vi "Get Sample Rate.vi"(8 "error in (no error)":errorcluster, 11 "Impulse Manager in":refnum<class "Impulse Manager.lvclass">) -> (0 "error out":errorcluster, 2 "Sample Rate":i32, 3 "Impulse Manager out":refnum<class "Impulse Manager.lvclass">)   [LabVIEW 2013, in "Impulse Manager.lvclass"]
uses:
  Impulse Manager.lvclass
  Impulse Manager.lvclass/Impulse Manager.ctl
  Impulse Data/Impulse Data.lvclass
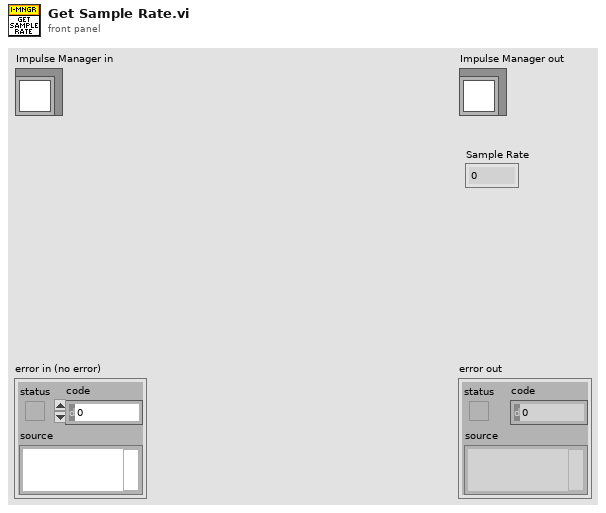
[diagram p1: front panel]
types:
  T1 = typedef "Impulse Data.lvclass/Instance handle.ctl" = refnum<data-value>
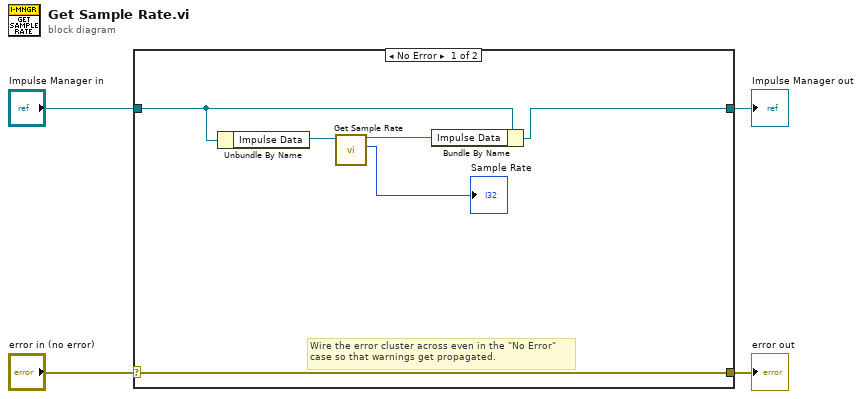
[diagram p0: block diagram]
diagram:
  n1 = case shown="No Error" "error in (no error)" {
    selector: "error in (no error)" -> [w10 w12]
    tunnel: [w10 w12] -> w3
    tunnel: [w7 w11] -> w1
    tunnel: "Impulse Manager in" -> [w8 w11]
    frame No Error {
      # "Wire the error cluster across even in the \"No Error\"\ncase so that warnings get propagated."
      n2 = Unbundle By Name(w8) -> ("Impulse Data"=w9:T1)
      n3 = call "Get Sample Rate.vi"("Reference in"=w9) -> ("Sample Rate"=→"Sample Rate":i32, "Reference out"=w6:T1)  [unwired: 8 in, 1 out]
      n4 = Bundle By Name(cluster=w8, "Impulse Data"=w6) -> (w7:refnum<class "Impulse Manager.lvclass">)
    }
    frame Error {
    }
  }
  "error out" <- w3
  "Impulse Manager out" <- w1
